vi "UDP接收测试.vi"() -> (2 "接收数据":string)   [LabVIEW 2010]
panel:
  out "数组 2":u16[](array[numeric]) format="%x"
  out "结束":bool
  in  "清除":bool
  out "数组":u8[](array[numeric]) format="%x"
  in  "停止":bool
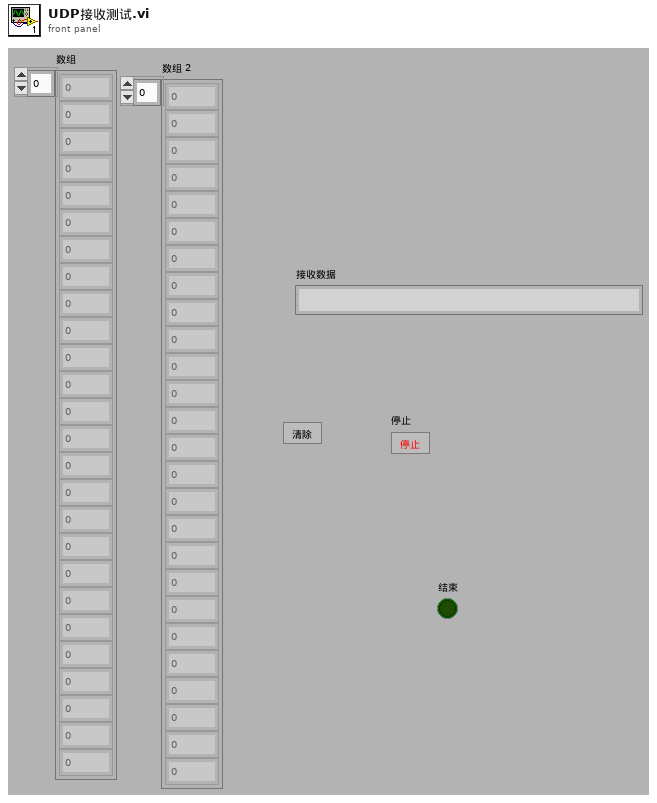
[diagram p1: front panel]
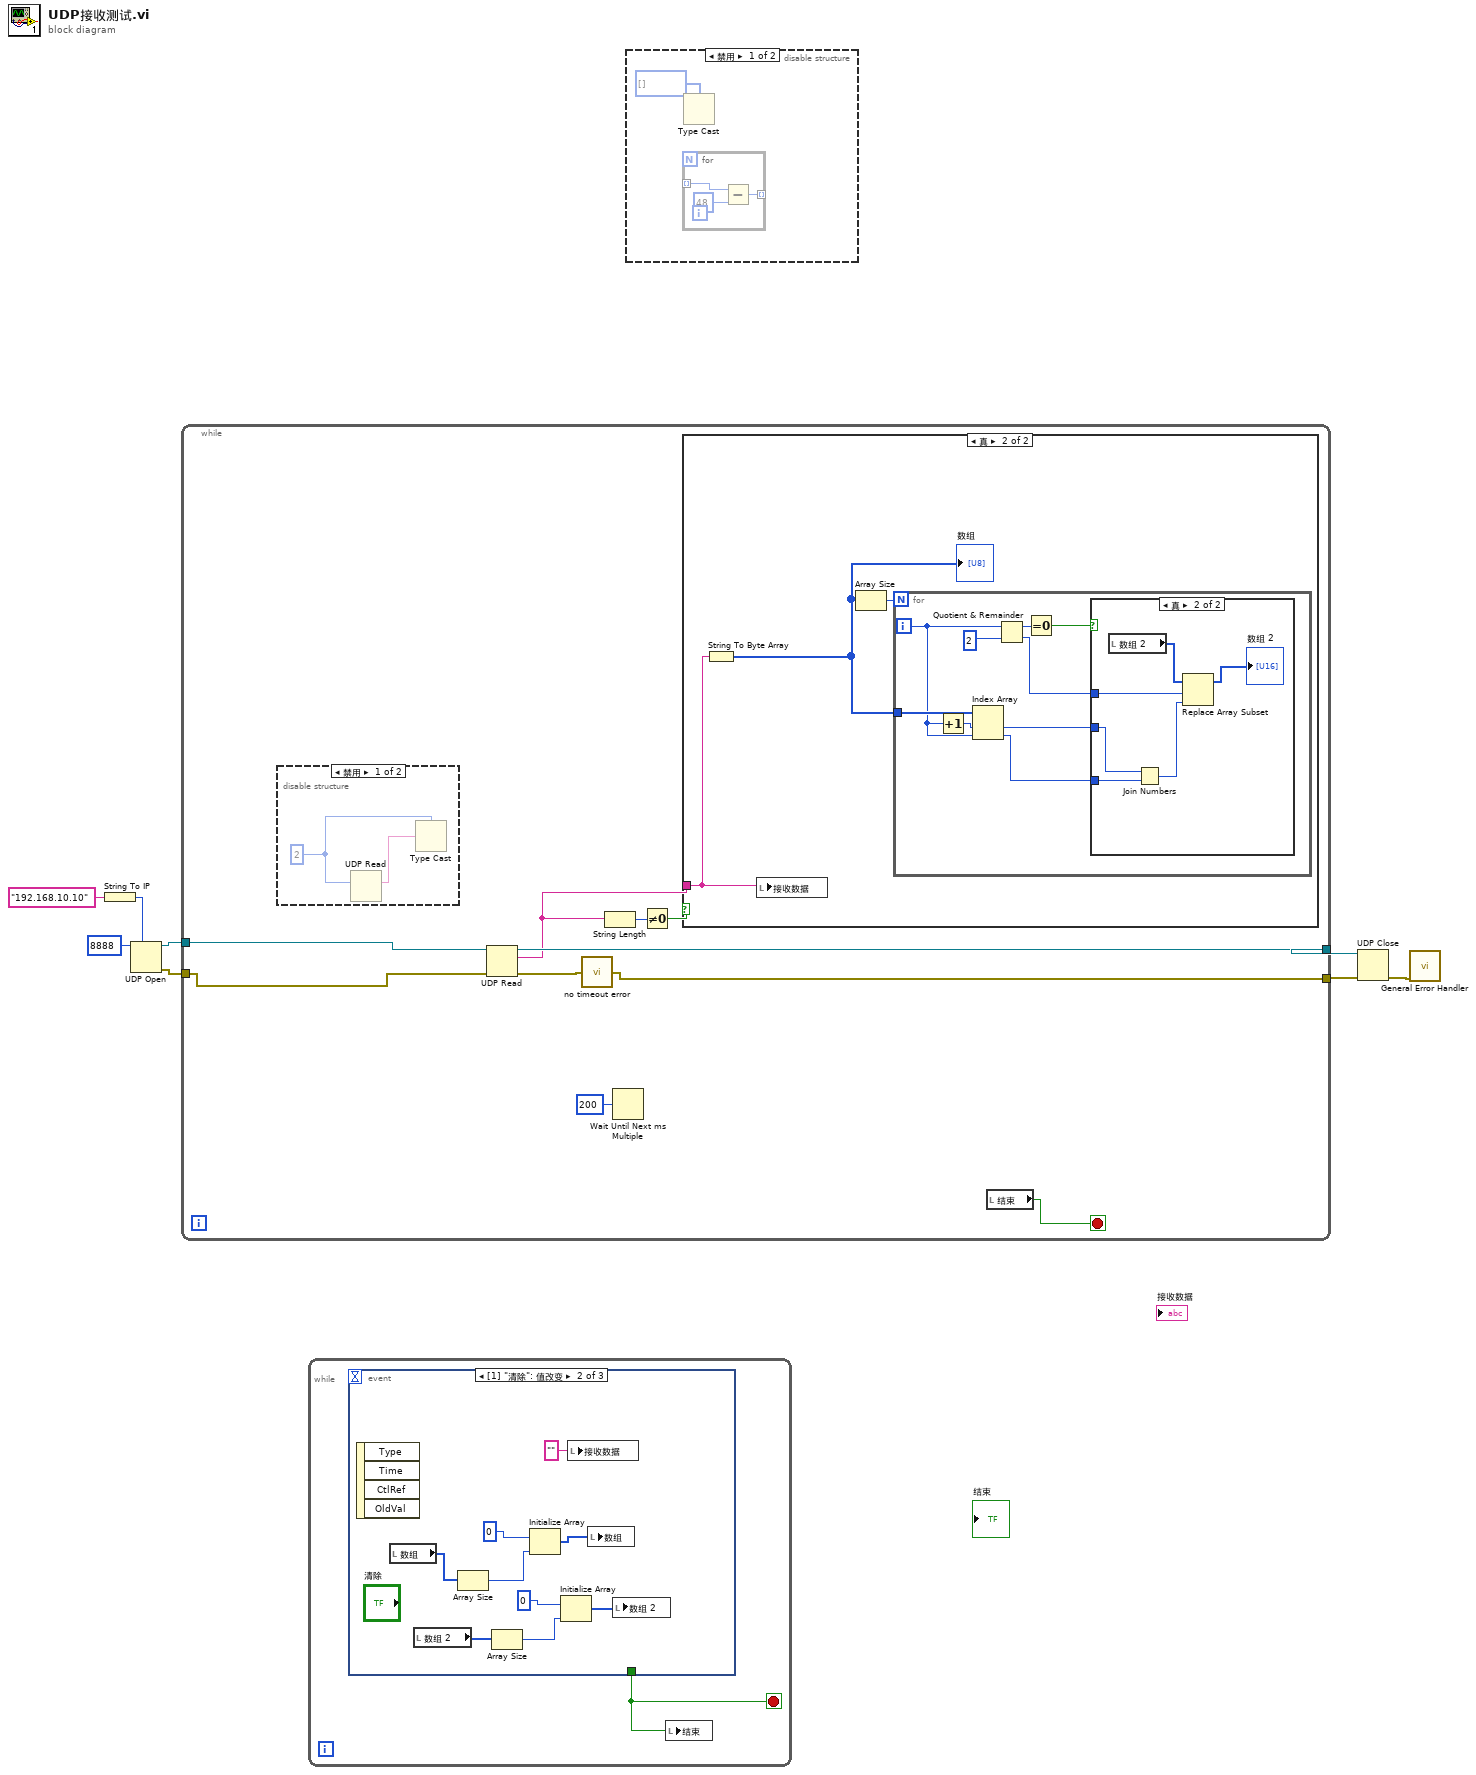
[diagram p0: block diagram]
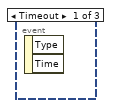
[diagram p3: hidden frame]
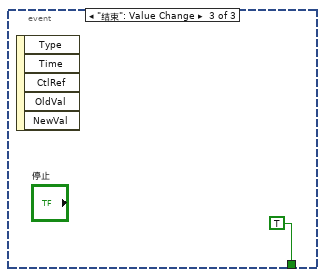
[diagram p4: hidden frame]
diagram:
  n1 = String To IP(1:"192.168.10.10" ("名称")) -> (0:w8:u32)
  n2 = UDP Open(7:w8, 11:u16 8888 ("端口")) -> (port=w7:refnum<k16>, 0:w6:errorcluster)  [unwired: 3 in, 1 out]
  n3 = while {
    tunnel: w7 -> [w10]
    tunnel: w6 -> [w9]
    tunnel: [w14] -> w4
    tunnel: [w13] -> w3
    stop <- w12 stop-if-true
    n4 = disable-structure shown="禁用" {
      frame Disabled {
        w19 = 2 ("最大值(548)")
        n5 = UDP Read(max size (548)=w19) -> (data out=w20:string)  [unwired: 3 in, 4 out]
        n6 = Type Cast(type=w19, x=w20) -> ()  [unwired: 1 out]
      }
      frame Enabled {
      }
    }
    n7 = UDP Read(connection ID=w10, 8:w9) -> (data out=w11:string, error out=w16:errorcluster, 3:w14:refnum<k16>)  [unwired: 2 in, 2 out]
    n8 = call "no timeout error.vi"("error in (no error)"=w16) -> ("error out"=w13:errorcluster)
    n9 = String Length(string=w11) -> (length=w18:i32)
    n10 = Wait Until Next ms Multiple(millisecond multiple=u32 200 ("毫秒倍数")) -> ()  [unwired: 1 out]
    n11 = Not Equal To 0?(x=w18) -> (x != 0?=w17:bool)
    n12 = case shown="真" w17 {
      tunnel: w11 -> [_ w22]
      frame False {
      }
      frame True {
        n13 = String To Byte Array(string=w22) -> (unsigned byte array=w21:u8[])
        "数组" <- w21
        n14 = local write "接收数据"(w22) -> ()
        n15 = Array Size(array=w21) -> (size(s)=w23:i32)
        n16 = for {
          N: w23 -> [_]
          tunnel: w21 -> [w29]
          i -> [w27]
          n17 = Increment(x=w27) -> (x+1=w28:i32)
          n18 = Index Array(array=w29, index #1=w28, index #2=w27) -> (element #1=w25:u8, element #2=w24:u8)
          n19 = Quotient & Remainder(x=w27, y=2) -> (x-y*floor(x/y)=w31:i32, floor(x/y)=w26:i32)
          n20 = Equal To 0?(x=w31) -> (x = 0?=w30:bool)
          n21 = case shown="真" w30 {
            tunnel: w26 -> [_ w36]
            tunnel: w25 -> [_ w34]
            tunnel: w24 -> [_ w33]
            frame False {
            }
            frame True {
              n22 = local read "数组 2"() -> (w38:u16[])
              n23 = Join Numbers(hi=w34, lo=w33) -> ((hi.lo)=w37:u16)
              n24 = Replace Array Subset(array=w38, new element=w37, index=w36) -> (→"数组 2":u16[])
            }
          }
        }
      }
    }
    n25 = local read "结束"() -> (w12:bool)
  }
  n26 = while {
    stop <- w39 stop-if-true
    n27 = event shown="[1] \"清除\": 值改变" {
      selector: _ -> [_ _ _]
      dyn-events: _ -> [_ _ _]
      timeout: _ -> [_ _ _]
      tunnel: [_ _ TRUE] -> w39
      event Timeout {
        n28 = event-data() -> ()  [unwired: 1 in, 2 out]
      }
      event "清除": Value Change {
        n29 = event-data() -> ()  [unwired: 1 in, 4 out]
        n30 = local read "数组"() -> (w45:u8[])
        n31 = local read "数组 2"() -> (w43:u16[])
        n32 = Array Size(array=w45) -> (size(s)=w44:i32)
        n33 = Array Size(array=w43) -> (size(s)=w41:i32)
        n34 = Initialize Array(u8 0, w44) -> (w47:u8[])
        n35 = Initialize Array(u16 0, w41) -> (w40:u16[])
        n36 = local write "接收数据"("" ("接收数据")) -> ()
        n37 = local write "数组"(w47) -> ()
        n38 = local write "数组 2"(w40) -> ()
      }
      event "结束": Value Change {
        n39 = event-data() -> ()  [unwired: 1 in, 5 out]
      }
    }
    n40 = local write "结束"(w39) -> ()
  }
  n41 = disable-structure shown="禁用" {
    frame Disabled {
      n42 = for {
        tunnel: _ -> [w52] mode=indexing
        tunnel: [w51] -> _ mode=indexing
        n43 = Subtract(x=w52, y=u8 48) -> (x-y=w51:u8)
      }
      n44 = Type Cast(type=u8[] []) -> ()  [unwired: 1 in, 1 out]
    }
    frame Enabled {
    }
  }
  n45 = UDP Close(connection ID=w4, 8:w3) -> (error out=w5:errorcluster)  [unwired: 1 out]
  n46 = call <vilib>:"General Error Handler.vi"("error in (no error)"=w5) -> ()  [unwired: 10 in, 5 out]
